vi "Initialize.vi"(8 "error in (no error)":errorcluster) -> (0 "error out":errorcluster, 3 "CIFChannelMng out":refnum<class "CIFChannelMng.lvclass">)   [LabVIEW 2021, in "CIFChannelMng.lvclass"]
uses:
  CIFChannelMng.lvclass
  CIFChannelMng.lvclass/CIFChannelMng.ctl
  <vilib>/CIF Foundation/CIF Channels Core/ChannelCommon/typedef/Channel Pattern.ctl
  <vilib>/CIF Foundation/CIF Channels Core/ChannelCommon/ChannelCommon.lvlib
  <vilib>/CIF Foundation/CIF Channels Core/ChannelCommon/typedef/Direction.ctl
  typedef/Channel List for OOB.ctl
  typedef/TX DVR Data.ctl
  typedef/TX Commands.ctl
  f6679ebb-52fd-4a94-bdae-d35de3237da0.vi
  typedef/FIFO Publisher Return.ctl
  typedef/TX CIPC Data.ctl
  <vilib>/CIF Foundation/CIF Channels Core/ChannelCommon/typedef/New FIFO Instance Response.ctl
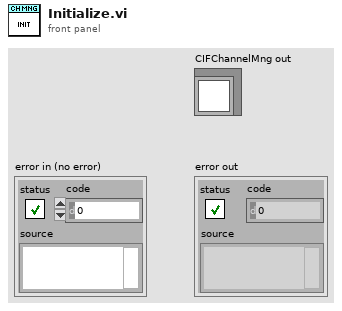
[diagram p1: front panel]
types:
  T1 = typedef "CIFChannelMng.lvclass/TX CIPC Data.ctl" = cluster{"TX Commands":T2}
  T2 = typedef "CIFChannelMng.lvclass/TX Commands.ctl" = enum8{"Channel List", "New FIFO Pub"}
  T3 = typedef "CIFChannelMng.lvclass/TX DVR Data.ctl" = cluster{"Channel List":T4[], "Publisher Instance":T7}
  T4 = typedef "CIFChannelMng.lvclass/Channel List for OOB.ctl" = cluster{"Name":string, "Direction":T5, "Type":string, "Connected?":bool, "Connected Name":string, "Custom Config Data":u8[], "Forced?":bool, "Pattern":T6}
  T5 = typedef "ChannelCommon.lvlib/Direction.ctl" = enum8{"Publisher", "Subscriber"}
  T6 = typedef "ChannelCommon.lvlib/Channel Pattern.ctl" = enum8{"Unknown", "Tag", "FIFO", "MultiFIFO", "BackpressureFIFO"}
  T7 = typedef "CIFChannelMng.lvclass/FIFO Publisher Return.ctl" = cluster{"FIFO Instance Config":T8, "error":errorcluster, "Added":bool}
  T8 = typedef "ChannelCommon.lvlib/New FIFO Instance Response.ctl" = cluster{"Publisher":string, "Custom Data":u8[]}
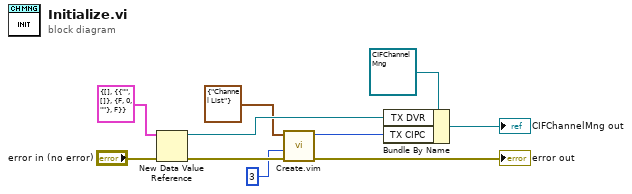
[diagram p0: block diagram]
diagram:
  n1 = New Data Value Reference(data value=T3 {"Channel List"=[], "Publisher Instance"={"FIFO Instance Config"={"Publisher"="", "Custom Data"=[]}, "error"={"status"=FALSE, "code"=0, "source"=""}, "Added"=FALSE}} ("Template Payload"), error in="error in (no error)") -> (data value reference=w7:refnum<data-value>, error out=w3:errorcluster)
  n2 = call "Create.vim"("error in (no error)"=w3, "Buffer Size N (2^N)"=u8 3, "Data Type"=T1 {"TX Commands"=enum."Channel List"}) -> ("error out"=→"error out":errorcluster, "CIPC Reference"=w5:u64)  [unwired: 5 in, 2 out]
  n3 = Bundle By Name(cluster=refnum<class "CIFChannelMng.lvclass"> refnum ("CIFChannelMng out"), "TX DVR"=w7, "TX CIPC"=w5) -> (→"CIFChannelMng out":refnum<class "CIFChannelMng.lvclass">)
